vi "_시리얼-패킷 데이타-전송.vi"(3 "전송 문자열":string="FPGARX 0 1", 4 "ID":u8 format="%02x", 5 "시리얼 포트":refnum<visa-resource-name>) -> (0 "Processing Time(ms)":u32, 2 "송신 실패(T)":bool)   [LabVIEW 2014]
panel:
  out "수신 문자열 버퍼":string
  out "수신 타이머 값":u32
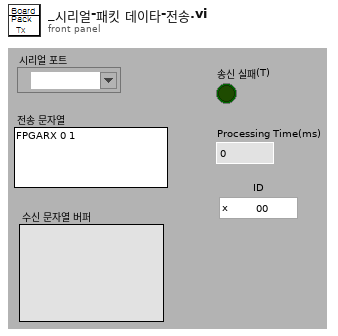
[diagram p1: front panel]
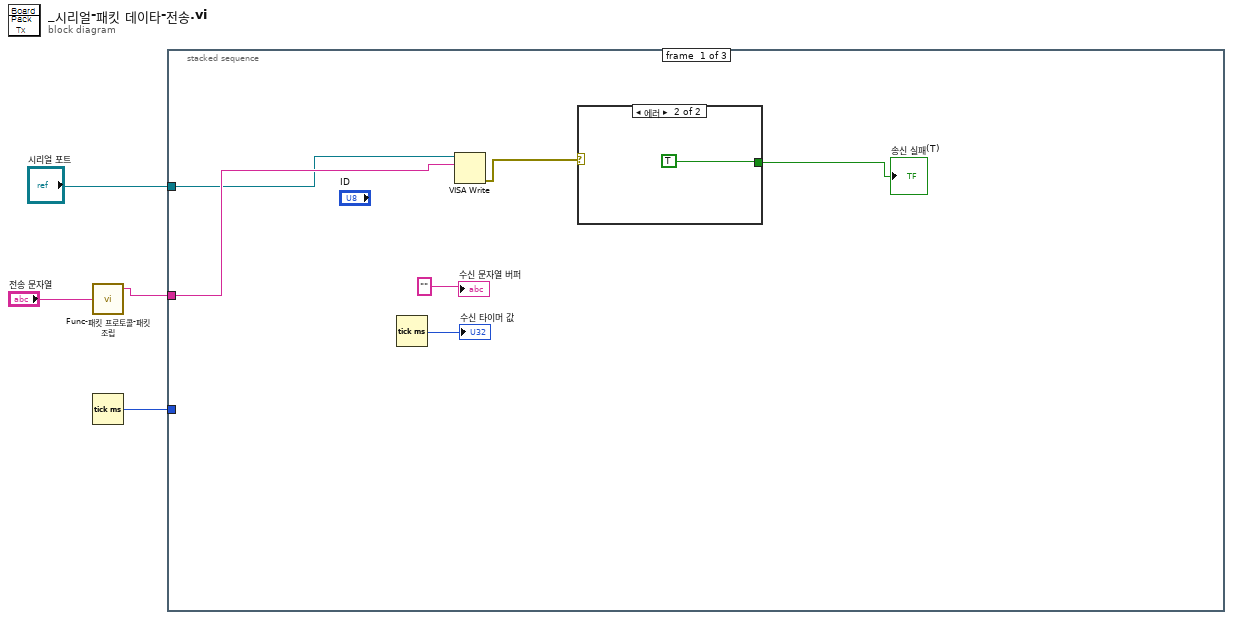
[diagram p0: block diagram]
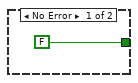
[diagram p2: hidden frame]
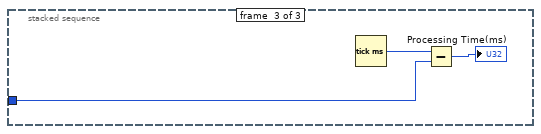
[diagram p4: hidden frame]
diagram:
  n1 = call "Func-패킷 프로토콜-패킷 조립.vi"("메시지 데이터"="전송 문자열") -> ("패킷 데이터 (Hex)"=w1:string)  [unwired: 4 in]
  n2 = Tick Count (ms)() -> (millisecond timer value=w3:u32)
  n3 = stacked-sequence {
    tunnel: "시리얼 포트" -> [w7 _ _]
    tunnel: w1 -> [w10 _ _]
    tunnel: w3 -> [_ _ w13]
    frame #0 {
      n4 = Tick Count (ms)() -> (millisecond timer value=→"수신 타이머 값":u32)
      n5 = VISA Write(VISA resource name=w7, write buffer=w10) -> (error out=w6:errorcluster)  [unwired: 1 in, 2 out]
      n6 = case shown="에러" w6 {
        tunnel: [FALSE TRUE] -> w5
        frame No Error {
        }
        frame Error {
        }
      }
      "송신 실패(T)" <- w5
      "수신 문자열 버퍼" <- "" ("수신 문자열 버퍼")
    }
    frame #1 {
    }
    frame #2 {
      n7 = Tick Count (ms)() -> (millisecond timer value=w15:u32)
      n8 = Subtract(x=w15, y=w13) -> (x-y=→"Processing Time(ms)":u32)
    }
  }
